vi "callingViReference.vi"() -> (0 "Caller's VI Reference":refnum<vi>)   [LabVIEW 2017, in "shared.lvlib"]
doc: "Returns a reference to the caller's VI."
uses:
  shared.lvlib
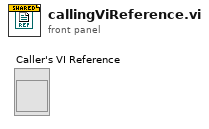
[diagram p1: front panel]
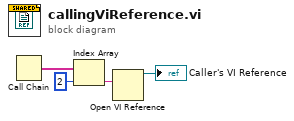
[diagram p0: block diagram]
diagram:
  n1 = Call Chain() -> (call chain=w3:string[])
  n2 = Index Array(array=w3, index=2) -> (element=w2:string)
  n3 = Open VI Reference(vi path=w2) -> (vi reference=→"Caller's VI Reference":refnum<vi>)  [unwired: 5 in, 1 out]
